vi "Start.vi"(8 "error in (no error)":errorcluster, 11 "DMM in":refnum<class "NI DMM.lvclass">) -> (0 "error out":errorcluster, 3 "DMM out":refnum<class "NI DMM.lvclass">)   [LabVIEW 2020, in "NI DMM.lvlib" / "NI DMM.lvclass"]
uses:
  NI DMM.lvclass
  NI DMM.lvclass/NI DMM.ctl
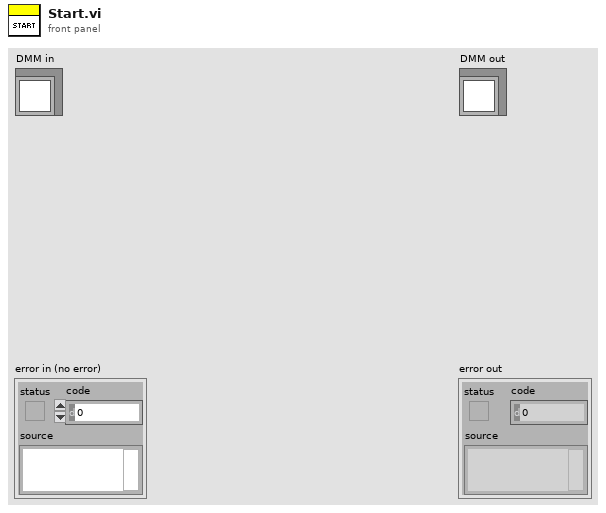
[diagram p1: front panel]
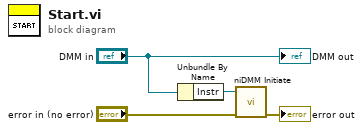
[diagram p0: block diagram]
diagram:
  n1 = Unbundle By Name("DMM in") -> ("Instr"=w3:refnum<k15>)
  n2 = call <instrlib>:"niDMM Initiate.vi"("error in (no error)"="error in (no error)", "instrument handle"=w3) -> ("error out"=→"error out":errorcluster)  [unwired: 8 in, 1 out]
  "DMM out" <- "DMM in"
